vi "测量系统.vi"() -> ()   [LabVIEW 2012]
uses:
  <vilib>/Platform/TimedLoop/XDataNode/timing_clust.ctl
  <vilib>/Platform/TimedLoop/XDataNode/nitl_modes.ctl
  <vilib>/Platform/TimedLoop/XDataNode/wakeup.ctl
  <vilib>/Instr/_visa.llb/VISA Configure Serial Port (Instr).vi
  <vilib>/Platform/TimedLoop/XDataNode/XDataNode.xnode
  <vilib>/Platform/TimedLoop/XDataNode/XDNodeRunTimeDep.lvlib
panel:
  in  "元素 5":i32
  in  "元素 4":i32
  in  "元素 3":i32
  in  "周期":i64
  in  "停止 2":bool
  in  "元素 2":i32
  in  "停止":bool
  in  "元素":i32
  out "当前湿度值":dbl(knob) scale=0.0..100.0
  out "当前温度值":dbl(knob) scale=0.0..100.0
  in  "串口号：":refnum<visa-resource-name>
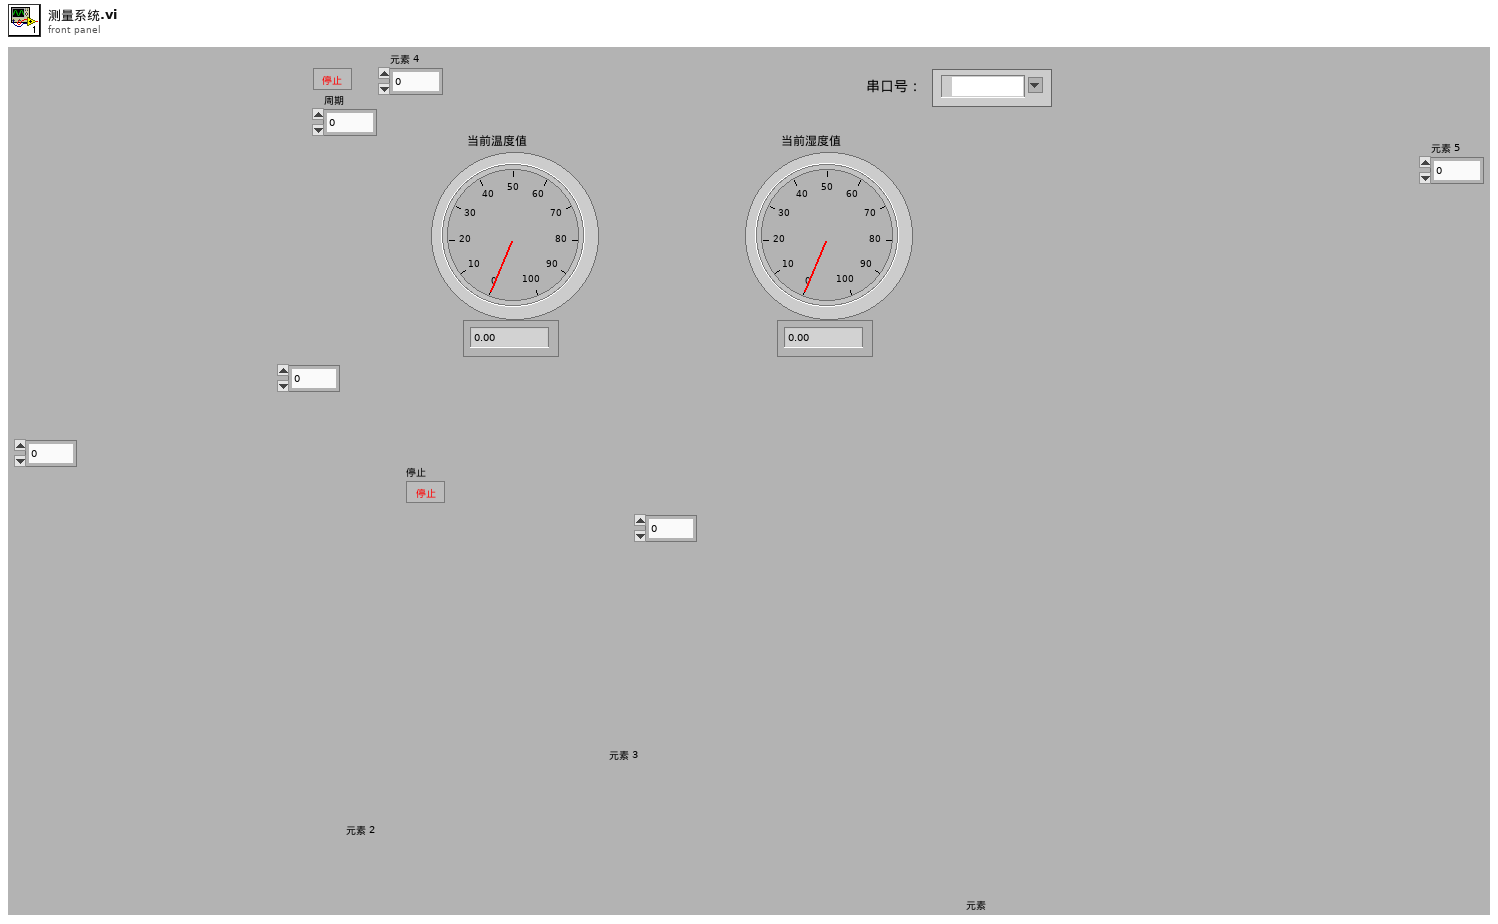
[diagram p1: front panel]
types:
  T1 = typedef "XDNodeRunTimeDep.lvlib/timing_clust.ctl" = cluster{"Expected End [f-1]":u64, "Actual End [f-1]":u64, "Finished Late? [f-1]":bool, "Expected End [i-1]":u64, "Actual End [i-1]":u64, "Finished Late? [i-1]":bool, "Expected Start [i]":u64, "Actual Start [i]":u64, "Expected Start [f]":u64, "Actual Start [f]":u64, "Source Name":string, "Structure Name":string, "Period":i64, "Deadline":i64, "Offset":i64, "Start":i64, "Priority":i32, "Timeout":i32, "Mode":T2, "Wakeup Reason":T3, "Error":errorcluster, "Source Type":string, "Secondary Source Type":string, "Global End Time":u64, "Global Start Time":u64, "Frame Duration":u64, "Iteration Duration":u64, "Assigned CPU":i32, "I/O Scan Engine Mode":u32}
  T2 = typedef "XDNodeRunTimeDep.lvlib/nitl_modes.ctl" = enum32{"No Change", "Process missed periods, maintain original phase", "Discard missed periods, maintain original phase", "Process missed periods, ignore original phase", "Discard missed periods, ignore original phase"}
  T3 = typedef "XDNodeRunTimeDep.lvlib/wakeup.ctl" = enum32{"Normal", "Aborted", "Asynchronous wakeup", "Timing source error", "Timed loop error", "Timeout"}
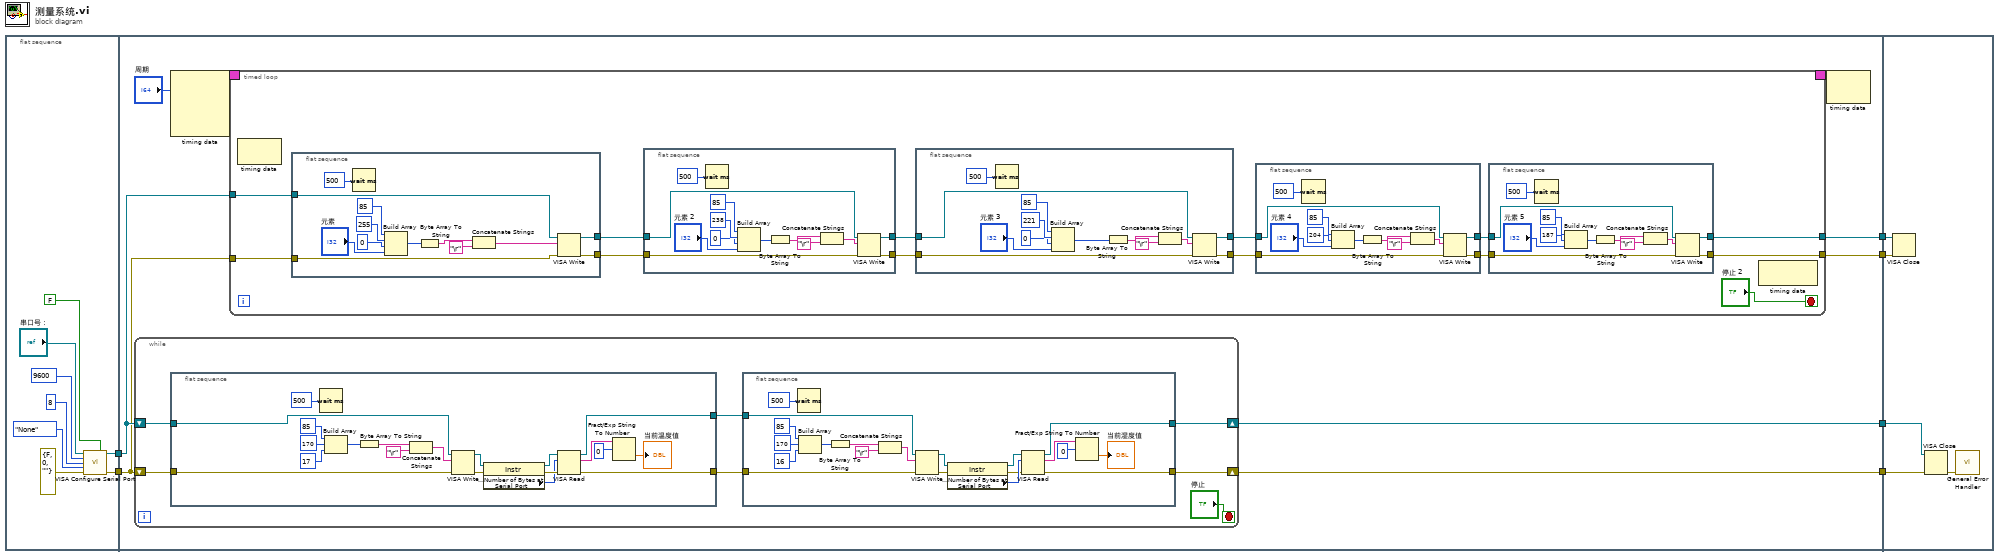
[diagram p0: block diagram]
diagram:
  n1 = flat-sequence {
    tunnel: [w9] -> w6
    tunnel: [w8] -> w5
    tunnel: w6 -> [w18]
    tunnel: w5 -> [w17]
    tunnel: [w23] -> w4
    tunnel: [w22] -> w3
    tunnel: [w16] -> w2
    tunnel: [w15] -> w1
    tunnel: w4 -> [w157]
    tunnel: w3 -> [w156]
    tunnel: w2 -> [w155]
    tunnel: w1 -> [w154]
    frame #0 {
      n2 = call-poly "VISA Configure Serial Port"("VISA resource name"="串口号：", "Enable Termination\nChar (T)"=FALSE ("Enable Termination\nChar (T)"), "baud rate (9600)"=u32 9600, "data bits (8)"=u16 8, "parity (0:none)"=enum16{"None", "Odd", "Even", "Mark", "Space"}."None", "error in (no error)"=errorcluster {"status"=FALSE, "code"=0, "source"=""}) -> ("VISA resource name out"=w9:refnum<visa-resource-name>, "error out"=w8:errorcluster)  [unwired: 1 in, 7 out]
    }
    frame #1 {
      n3 = while {
        shift-right: [w110] -> w22
        shift-left: w17 -> [w106]
        shift-right: [w109] -> w23
        shift-left: w18 -> [w107]
        stop <- "停止" stop-if-true
        n4 = flat-sequence {
          tunnel: w107 -> [w152]
          tunnel: w106 -> [w151]
          tunnel: [w133] -> w112
          tunnel: [w134] -> w111
          frame #0 {
            n5 = Wait (ms)(milliseconds to wait=u32 500 ("等待时间（毫秒）")) -> ()  [unwired: 1 out]
            n6 = Build Array(85, 170, 17) -> (w149:i32[])
            n7 = Byte Array To String(unsigned byte array=w149) -> (string=w144:string)
            n8 = Concatenate Strings(w144, "\r") -> (w145:string)
            n9 = VISA Write(VISA resource name=w152, write buffer=w145, error in (no error)=w151) -> (VISA resource name out=w140:refnum<visa-resource-name>, error out=w139:errorcluster)  [unwired: 1 out]
            n10 = property class="Instr"(reference=w140, error in=w139) -> (reference out=w138:refnum<visa-resource-name>, error out=w137:errorcluster, "Serial Settings:Number of Bytes at Serial Port"=w136:u32)
            n11 = VISA Read(VISA resource name=w138, byte count=w136, error in (no error)=w137) -> (VISA resource name out=w133:refnum<visa-resource-name>, read buffer=w142:string, error out=w134:errorcluster)  [unwired: 1 out]
            n12 = Fract/Exp String To Number(string=w142, offset=0 ("偏移量")) -> (number=→"当前温度值":dbl)  [unwired: 2 in, 1 out]
          }
        }
        n13 = flat-sequence {
          tunnel: [w113] -> w109
          tunnel: w112 -> [w116]
          tunnel: [w115] -> w110
          tunnel: w111 -> [w114]
          frame #0 {
            n14 = Wait (ms)(milliseconds to wait=u32 500 ("等待时间（毫秒）")) -> ()  [unwired: 1 out]
            n15 = Build Array(85, 170, 16) -> (w118:i32[])
            n16 = Byte Array To String(unsigned byte array=w118) -> (string=w123:string)
            n17 = Concatenate Strings(w123, "\r") -> (w122:string)
            n18 = VISA Write(VISA resource name=w116, write buffer=w122, error in (no error)=w114) -> (VISA resource name out=w127:refnum<visa-resource-name>, error out=w128:errorcluster)  [unwired: 1 out]
            n19 = property class="Instr"(reference=w127, error in=w128) -> (reference out=w129:refnum<visa-resource-name>, error out=w130:errorcluster, "Serial Settings:Number of Bytes at Serial Port"=w131:u32)
            n20 = VISA Read(VISA resource name=w129, byte count=w131, error in (no error)=w130) -> (VISA resource name out=w113:refnum<visa-resource-name>, read buffer=w125:string, error out=w115:errorcluster)  [unwired: 1 out]
            n21 = Fract/Exp String To Number(string=w125, offset=0 ("偏移量")) -> (number=→"当前湿度值":dbl)  [unwired: 2 in, 1 out]
          }
        }
      }
      n22 = node-c288("周期") -> (w21:T1)  [unwired: 3 in]
      n23 = timed-loop {
        timing: w21 -> [_]
        timing-out: [_] -> w20
        tunnel: w18 -> [w35]
        tunnel: w17 -> [w34]
        tunnel: [w25] -> w16
        tunnel: [w24] -> w15
        stop <- "停止 2" stop-if-true
        n24 = node-c288() -> ()  [unwired: 1 in, 1 out]
        n25 = flat-sequence {
          tunnel: [w94] -> w33
          tunnel: [w93] -> w32
          tunnel: w35 -> [w90]
          tunnel: w34 -> [w89]
          frame #0 {
            n26 = Wait (ms)(milliseconds to wait=u32 500 ("等待时间（毫秒）")) -> ()  [unwired: 1 out]
            n27 = Build Array(85, 255, 0 ("元素"), "元素") -> (w96:i32[])
            n28 = Byte Array To String(unsigned byte array=w96) -> (string=w101:string)
            n29 = Concatenate Strings(w101, "\r") -> (w100:string)
            n30 = VISA Write(VISA resource name=w90, write buffer=w100, error in (no error)=w89) -> (VISA resource name out=w94:refnum<visa-resource-name>, error out=w93:errorcluster)  [unwired: 1 out]
          }
        }
        n31 = flat-sequence {
          tunnel: [w81] -> w31
          tunnel: [w80] -> w30
          tunnel: w33 -> [w77]
          tunnel: w32 -> [w76]
          frame #0 {
            n32 = Wait (ms)(milliseconds to wait=u32 500 ("等待时间（毫秒）")) -> ()  [unwired: 1 out]
            n33 = Build Array(85, 238, 0 ("元素"), "元素 2") -> (w83:i32[])
            n34 = Byte Array To String(unsigned byte array=w83) -> (string=w88:string)
            n35 = Concatenate Strings(w88, "\r") -> (w87:string)
            n36 = VISA Write(VISA resource name=w77, write buffer=w87, error in (no error)=w76) -> (VISA resource name out=w81:refnum<visa-resource-name>, error out=w80:errorcluster)  [unwired: 1 out]
          }
        }
        n37 = flat-sequence {
          tunnel: [w66] -> w28
          tunnel: [w65] -> w29
          tunnel: w31 -> [w62]
          tunnel: w30 -> [w61]
          frame #0 {
            n38 = Wait (ms)(milliseconds to wait=u32 500 ("等待时间（毫秒）")) -> ()  [unwired: 1 out]
            n39 = Build Array(85, 221, 0 ("元素"), "元素 3") -> (w68:i32[])
            n40 = Byte Array To String(unsigned byte array=w68) -> (string=w73:string)
            n41 = Concatenate Strings(w73, "\r") -> (w72:string)
            n42 = VISA Write(VISA resource name=w62, write buffer=w72, error in (no error)=w61) -> (VISA resource name out=w66:refnum<visa-resource-name>, error out=w65:errorcluster)  [unwired: 1 out]
          }
        }
        n43 = flat-sequence {
          tunnel: [w54] -> w27
          tunnel: [w53] -> w26
          tunnel: w28 -> [w51]
          tunnel: w29 -> [w50]
          frame #0 {
            n44 = Wait (ms)(milliseconds to wait=u32 500 ("等待时间（毫秒）")) -> ()  [unwired: 1 out]
            n45 = Build Array(85, 204, "元素 4") -> (w55:i32[])
            n46 = Byte Array To String(unsigned byte array=w55) -> (string=w60:string)
            n47 = Concatenate Strings(w60, "\r") -> (w59:string)
            n48 = VISA Write(VISA resource name=w51, write buffer=w59, error in (no error)=w50) -> (VISA resource name out=w54:refnum<visa-resource-name>, error out=w53:errorcluster)  [unwired: 1 out]
          }
        }
        n49 = flat-sequence {
          tunnel: [w42] -> w25
          tunnel: [w41] -> w24
          tunnel: w27 -> [w39]
          tunnel: w26 -> [w38]
          frame #0 {
            n50 = Wait (ms)(milliseconds to wait=u32 500 ("等待时间（毫秒）")) -> ()  [unwired: 1 out]
            n51 = Build Array(85, 187, "元素 5") -> (w43:i32[])
            n52 = Byte Array To String(unsigned byte array=w43) -> (string=w48:string)
            n53 = Concatenate Strings(w48, "\r") -> (w47:string)
            n54 = VISA Write(VISA resource name=w39, write buffer=w47, error in (no error)=w38) -> (VISA resource name out=w42:refnum<visa-resource-name>, error out=w41:errorcluster)  [unwired: 1 out]
          }
        }
        n55 = node-c288() -> ()  [unwired: 1 in, 1 out]
      }
      n56 = node-c288(w20) -> ()  [unwired: 1 out]
    }
    frame #2 {
      n57 = VISA Close(VISA resource name=w155, error in (no error)=w154) -> ()  [unwired: 1 out]
      n58 = VISA Close(VISA resource name=w157, error in (no error)=w156) -> (error out=w153:errorcluster)
      n59 = call <vilib>:"General Error Handler.vi"("error in (no error)"=w153) -> ()  [unwired: 10 in, 5 out]
    }
  }
